vi "Stimulus.GetStatus.vi"(8 "error in (no error)":errorcluster, 11 "Cluster":T1) -> (0 "error out":errorcluster, 3 "cluster":T11)   [LabVIEW 2015, in "Single Station Execution.lvlib"]
uses:
  Single Station Execution.lvlib
  Types/Stimulus.Status.ctl
  Types/Execution.SequenceState.ctl
  Types/Main.StateVariables.ctl
  Types/INI.Settings.ctl
  <vilib>/NI Veristand/Execution/AlarmManager/AlarmManagerAPI.ctl
  NationalInstruments.VeriStand.ClientAPI
  <vilib>/NI Veristand/Execution/DataLogging/IDataLogging Ref.ctl
  <vilib>/NI Veristand/Execution/DataLogging/DataLoggingSpecification Ref.ctl
  Types/Execute.UserEventRefs.ctl
  <vilib>/NI Veristand/Execution/Workspace/SystemStateRegEventRef.ctl
  <vilib>/NI Veristand/Execution/Workspace/Target State Info.ctl
  <vilib>/NI Veristand/Execution/Workspace/Target State.ctl
  NationalInstruments.VeriStand.RealTimeSequenceDefinitionApi
  <vilib>/NI Veristand/Execution/Workspace/SystemStateEventRef.ctl
  <vilib>/NI Veristand/Execution/Workspace/WorkspaceAPI.ctl
  Types/UDPEngine.QueueCluster.ctl
  Types/UDPEngine.State.ctl
  <vilib>/NI Veristand/Execution/AlarmManager/NI_VS AlarmManager ExecutionAPI.lvlib
  <vilib>/NI Veristand/Execution/Workspace/NI_VS Workspace ExecutionAPI.lvlib
  <vilib>/NI Veristand/Execution/DataLogging/NI_VS Data Logging API.lvlib
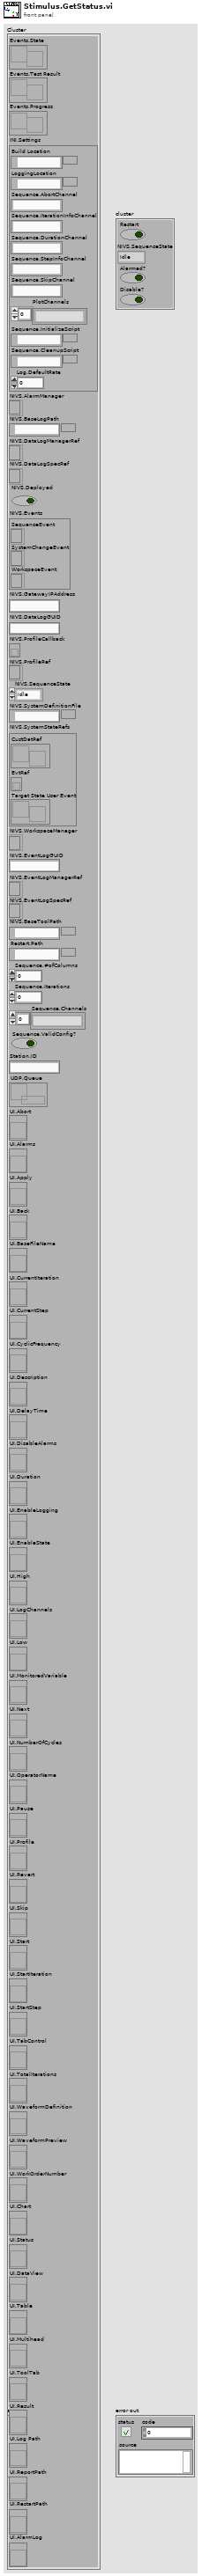
[diagram p1: front panel]
types:
  T1 = typedef "Single Station Execution.lvlib/Main.StateVariables.ctl" = cluster{"Events.State":refnum<user-event>, "Events.Test Result":refnum<user-event>, "Events.Progress":refnum<user-event>, "INI.Settings":T2, "NIVS.AlarmManager":T3, "NIVS.BaseLogPath":path, "NIVS.DataLogManagerRef":T4, "NIVS.DataLogSpecRef":T5, "NIVS.Deployed":bool, "NIVS.Events":T6, "NIVS.GatewayIPAddress":string, "NIVS.DataLogGUID":string, "NIVS.ProfileCallback":refnum<k27>, "NIVS.ProfileRef":refnum<k24>, "NIVS.SequenceState":T8, "NIVS.SystemDefinitionFile":path, "NIVS.SystemStateRefs":T9, "NIVS.WorkspaceManager":T10, "NIVS.EventLogGUID":string, "NIVS.EventLogManagerRef":T4, "NIVS.EventLogSpecRef":T5, "NIVS.BaseToolPath":path, "Restart.Path":path, "Sequence.#ofColumns":i32, "Sequence.Iterations":u32, "Sequence.Channels":string[], "Sequence.ValidConfig?":bool, "Station.ID":string, "UDP.Queue":refnum<queue>, "UI.Abort":refnum<vi>, "UI.Alarms":refnum<vi>, "UI.Apply":refnum<vi>, "UI.Back":refnum<vi>, "UI.BaseFileName":refnum<vi>, "UI.CurrentIteration":refnum<vi>, "UI.CurrentStep":refnum<vi>, "UI.CyclicFrequency":refnum<vi>, "UI.Description":refnum<vi>, "UI.DelayTime":refnum<vi>, "UI.DisableAlarms":refnum<vi>, "UI.Duration":refnum<vi>, "UI.EnableLogging":refnum<vi>, "UI.EnableState":refnum<vi>, "UI.High":refnum<vi>, "UI.LogChannels":refnum<vi>, "UI.Low":refnum<vi>, "UI.MonitoredVariable":refnum<vi>, "UI.Next":refnum<vi>, "UI.NumberOfCycles":refnum<vi>, "UI.OperatorName":refnum<vi>, "UI.Pause":refnum<vi>, "UI.Profile":refnum<vi>, "UI.Revert":refnum<vi>, "UI.Skip":refnum<vi>, "UI.Start":refnum<vi>, "UI.StartIteration":refnum<vi>, "UI.StartStep":refnum<vi>, "UI.TabControl":refnum<vi>, "UI.TotalIterations":refnum<vi>, "UI.WaveformDefinition":refnum<vi>, "UI.WaveformPreview":refnum<vi>, "UI.WorkOrderNumber":refnum<vi>, "UI.Chart":refnum<vi>, "UI.Status":refnum<vi>, "UI.DataView":refnum<vi>, "UI.Table":refnum<vi>, "UI.Multihead":refnum<vi>, "UI.ToolTab":refnum<vi>, "UI.Result":refnum<vi>, "UI.Log Path":refnum<vi>, "UI.ReportPath":refnum<vi>, "UI.RestartPath":refnum<vi>, "UI.AlarmLog":refnum<vi>}
  T2 = typedef "Single Station Execution.lvlib/INI.Settings.ctl" = cluster{"Build Location":path, "LoggingLocation":path, "Sequence.AbortChannel":string, "Sequence.IterationInfoChannel":string, "Sequence.DurationChannel":string, "Sequence.StepInfoChannel":string, "Sequence.SkipChannel":string, "PlotChannels":string[], "Sequence.InitializeScript":path, "Sequence.CleanupScript":path, "Log.DefaultRate":dbl}
  T3 = typedef "NI_VS AlarmManager ExecutionAPI.lvlib/AlarmManagerAPI.ctl" = refnum<k24>
  T4 = typedef "NI_VS Data Logging API.lvlib/IDataLogging Ref.ctl" = refnum<k24>
  T5 = typedef "NI_VS Data Logging API.lvlib/DataLoggingSpecification Ref.ctl" = refnum<k24>
  T6 = typedef "Single Station Execution.lvlib/Execute.UserEventRefs.ctl" = cluster{"SequenceEvent":refnum<event-registration>, "SystemChangeEvent":T7, "WorkspaceEvent":refnum<event-registration>}
  T7 = typedef "NI_VS Workspace ExecutionAPI.lvlib/SystemStateRegEventRef.ctl" = refnum<event-registration>
  T8 = typedef "Single Station Execution.lvlib/Execution.SequenceState.ctl" = enum16{"Idle", "Initializing", "Running", "Paused", "Finalizing", "Complete"}
  T9 = typedef "NI_VS Workspace ExecutionAPI.lvlib/SystemStateEventRef.ctl" = cluster{"CustDatRef":refnum<user-event>, "EvtRef":refnum<k27>, "Target State User Event":refnum<user-event>}
  T10 = typedef "NI_VS Workspace ExecutionAPI.lvlib/WorkspaceAPI.ctl" = refnum<k24>
  T11 = typedef "Single Station Execution.lvlib/Stimulus.Status.ctl" = cluster{"Restart":bool, "NIVS.SequenceState":T8, "Alarmed?":bool, "Disable?":bool}
  T12 = enum16{"Disabled", "Enabled", "Tripped", "Delayed Trip", "Indicate"}
  T13 = typedef "NI_VS Alarm ExecutionAPI.lvlib/AlarmInfo.ctl" = cluster{"Watch Channel":string, "High Limit Constant":bool, "High Limit Channel":string, "High Limit":dbl, "Low Limit Constant":bool, "Low Limit Channel":string, "Low Limit":dbl, "Procedure Name":string, "Delay":dbl, "Trip Value":dbl, "Priority":enum16{"Low", "Medium", "High"}, "State":enum16{"Disabled", "Enabled", "Tripped", "Delayed Trip", "Indicate"}, "Mode":enum16{"Normal", "Indicate Only"}, "Group Number":u32, "Priority Number":u32, "Name":string, "Full Name":string}
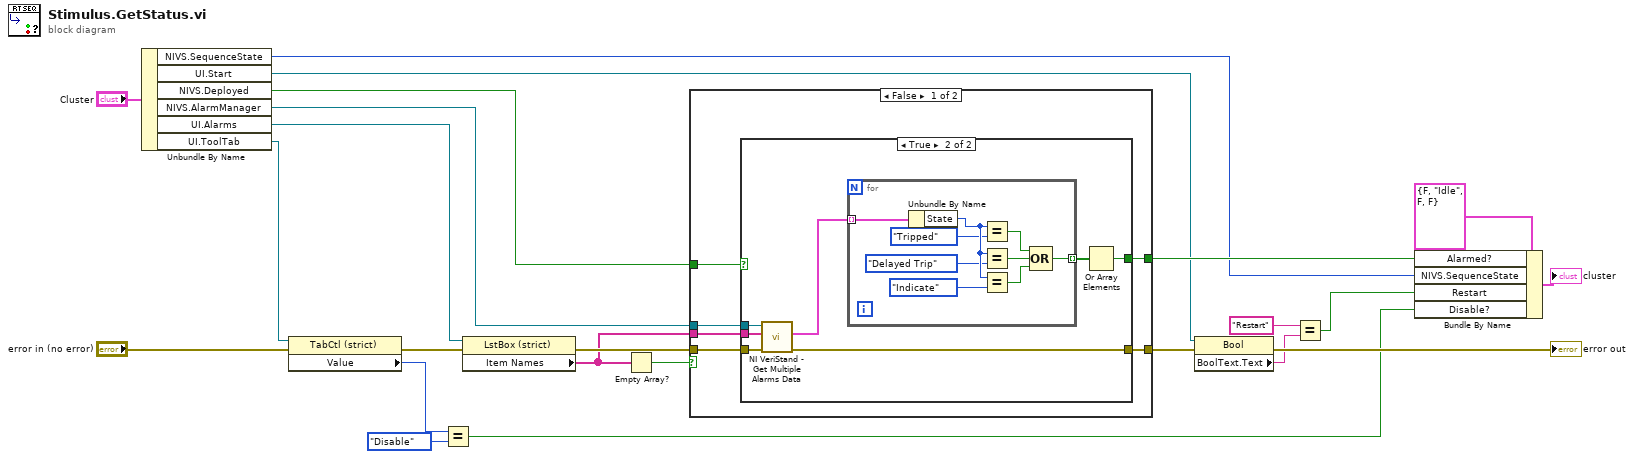
[diagram p0: block diagram]
diagram:
  n1 = Unbundle By Name("Cluster") -> ("NIVS.SequenceState"=w17:T8, "UI.Start"=w16:refnum<vi>, "NIVS.Deployed"=w7:bool, "NIVS.AlarmManager"=w10:T3, "UI.Alarms"=w11:refnum<vi>, "UI.ToolTab"=w6:refnum<vi>)
  n2 = property class="TabCtl (strict)"(reference=w6, error in="error in (no error)") -> (error out=w4:errorcluster, "Value"=w3:enum32{"Enable", "Disable"})  [unwired: 1 out]
  n3 = Equal?(x=w3, y=enum32{"Enable", "Disable"}."Disable") -> (x = y?=w1:bool)
  n4 = property class="LstBox (strict)"(reference=w11, error in=w4) -> (error out=w21:errorcluster, "Item Names"=w9:string[])  [unwired: 1 out]
  n5 = Empty Array?(array=w9) -> (empty?=w8:bool)
  n6 = case shown="False" w8 {
    tunnel: [w29 _] -> w23
    tunnel: [w28 w47] -> w22
    tunnel: w21 -> [w27 w47]
    tunnel: w9 -> [w26 _]
    tunnel: w10 -> [w25 _]
    tunnel: w7 -> [w24 _]
    frame False {
      n7 = case shown="True" w24 {
        tunnel: [_ w37] -> w29
        tunnel: [w30 w36] -> w28
        tunnel: w27 -> [w30 w35]
        tunnel: w26 -> [_ w34]
        tunnel: w25 -> [_ w31]
        frame False {
        }
        frame True {
          n8 = call <vilib>:"NI VeriStand - Get Multiple Alarms Data.vi"("error in (no error)"=w35, "Alarm Names"=w34, "AlarmManager in"=w31) -> ("error out"=w36:errorcluster, "Alarms Data"=w32:T13[])  [unwired: 6 in, 1 out]
          n9 = for {
            tunnel: [w39] -> w33 mode=indexing
            tunnel: w32 -> [w38] mode=indexing
            n10 = Unbundle By Name(w38) -> ("State"=w43:T12)
            n11 = Equal?(x=w43, y=T12."Tripped") -> (x = y?=w44:bool)
            n12 = Equal?(x=w43, y=T12."Delayed Trip") -> (x = y?=w45:bool)
            n13 = Equal?(x=w43, y=T12."Indicate") -> (x = y?=w46:bool)
            n14 = Compound Arithmetic op=OR(w44, w45, w46) -> (w39:bool)
          }
          n15 = Or Array Elements(Boolean array=w33) -> (logical OR=w37:bool)
        }
      }
    }
    frame True {
    }
  }
  n16 = property class="Bool"(reference=w16, error in=w22) -> (error out=→"error out":errorcluster, "BoolText.Text"=w13:string)  [unwired: 1 out]
  n17 = Equal?(x="Restart", y=w13) -> (x = y?=w20:bool)
  n18 = Bundle By Name(cluster=T11 {"Restart"=FALSE, "NIVS.SequenceState"=enum."Idle", "Alarmed?"=FALSE, "Disable?"=FALSE}, "Alarmed?"=w23, "NIVS.SequenceState"=w17, "Restart"=w20, "Disable?"=w1) -> (→"cluster":T11)
